vi "test SP Limiter.vi"() -> ()   [LabVIEW 2019]
uses:
  Reg/ctl/SpLim_State.ctl
  Reg/PID/PID SP Limiter/PID SP Limiter.lvclass
  Reg/PID/PID SP Limiter/PID SP Limiter.lvclass/PID SP Limiter.ctl
  Reg/control.lvlib
panel:
  in  "stop":bool
  out "pid_out_H":dbl format="%.2f"
  out "output":dbl format="%.2f"
  out "SpLim_State changed":bool
  out "dt (s) out":dbl
  in  "SP":dbl format="%#_13g"
  in  "SpLim_State":T1
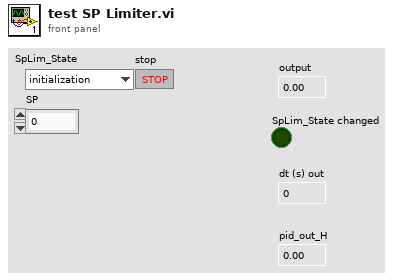
[diagram p1: front panel]
types:
  T1 = typedef "control.lvlib/SpLim_State.ctl" = enum8{"initialization", "stop", "decrease", "increase"}
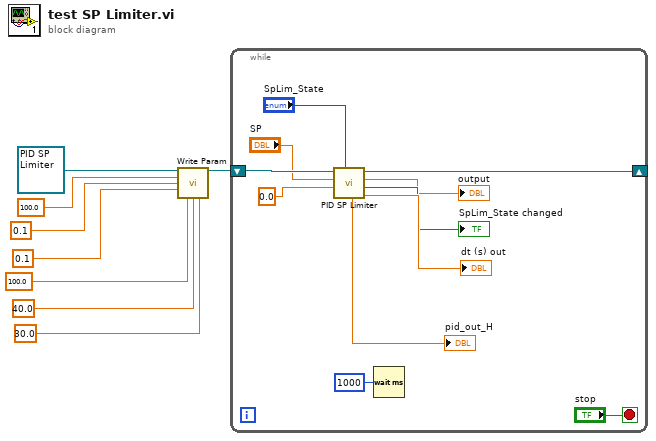
[diagram p0: block diagram]
diagram:
  n1 = call "Write Param.vi"("PID SP Limiter in"=refnum<class "PID SP Limiter.lvclass"> refnum, "SP_max"=100.0, "SP_start_rate"=0.1, "SP_stop_rate"=0.1, "Out_H"=100.0, "Out_start_H"=40.0, "Out_stop_H"=30.0) -> ("PID SP Limiter out"=w7:refnum<class "PID SP Limiter.lvclass">)  [unwired: 8 in]
  n2 = while {
    shift-right: [w11] -> _
    shift-left: w7 -> [w19]
    stop <- "stop" stop-if-true
    n3 = call "PID SP Limiter.vi"("SpLim_State"="SpLim_State", "PV"=0.0, "SP"="SP", "PID SP Limiter in"=w19) -> ("dt (s) out"=→"dt (s) out":dbl, "SpLim_State changed"=→"SpLim_State changed":bool, "output"=→"output":dbl, "PID SP Limiter out"=w11:refnum<class "PID SP Limiter.lvclass">, "pid_out_H"=→"pid_out_H":dbl)  [unwired: 3 in]
    n4 = Wait (ms)(milliseconds to wait=u32 1000) -> ()  [unwired: 1 out]
  }
